vi "test Get and Set RX Start Time.vi"(8 "error in (no error)":errorcluster, 11 "TestCase in":refnum<class "Framework Status Tests.lvclass">) -> (0 "error out":errorcluster, 3 "TestCase out":refnum<class "Framework Status Tests.lvclass">)   [LabVIEW 2017, in "Framework Status Tests.lvclass"]
uses:
  Framework Status Tests.lvclass
  Engine/Classes/Status/Framework Performance.lvclass/Framework Performance.ctl
  <vilib>/addons/_JKI Toolkits/VI Tester/TestCase.llb/TestCase.lvclass
  Engine/Classes/Status/Framework Performance.lvclass
  C:/Program Files (x86)/National Instruments/LabVIEW 2017/vi.lib/addons/_JKI Toolkits/VI Tester/TestCase.llb/TestCase.lvclass
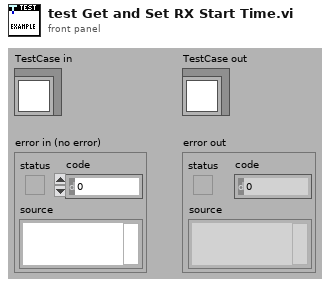
[diagram p1: front panel]
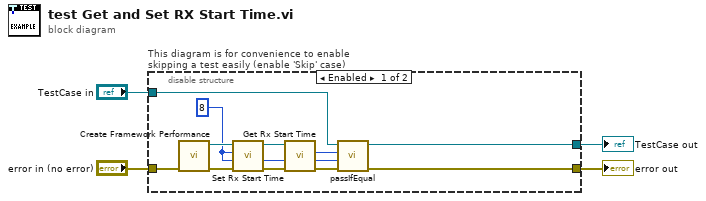
[diagram p0: block diagram]
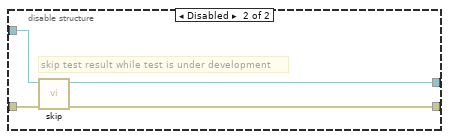
[diagram p2: hidden frame]
diagram:
  n1 = disable-structure "This diagram is for convenience to enable skipping a test easily (enable 'Skip' case)" shown="Enabled" {
    disable-tunnel: "TestCase in" -> [w11 w17]
    disable-tunnel: [w5 w15] -> w1
    disable-tunnel: [w6 w16] -> w3
    disable-tunnel: "error in (no error)" -> [w10 w14]
    frame Enabled {
      w7 = u32 8 ("Rx start time")
      n2 = call "Create Framework Performance.vi"("error in (no error)"=w10) -> ("error out"=w9:errorcluster, "Framework Performance"=w13:refnum<class "Framework Performance.lvclass">)  [unwired: 9 in]
      n3 = call "Set Rx Start Time.vi"("Rx start time"=w7, "Framework Performance in"=w13) -> ("Framework Performance out"=w12:refnum<class "Framework Performance.lvclass">)  [unwired: 9 in]
      n4 = call "Get Rx Start Time.vi"("Framework Performance in"=w12) -> ("Rx start time"=w8:u32)  [unwired: 9 in, 1 out]
      n5 = call-dynamic "passIfEqual.vi"("error in (no error)"=w9, "y"=w7, "x"=w8, "TestCase in"=w11) -> ("error out"=w6:errorcluster, "TestCase out"=w5:refnum<class "Framework Status Tests.lvclass">)  [unwired: 6 in]
    }
    frame Disabled {
      # "skip test result while test is under development"
      n6 = call <vilib>:"skip.vi"("error in (no error)"=w14, "TestCase in"=w17) -> ("error out"=w16:errorcluster, "TestCase out"=w15:refnum<class "Framework Status Tests.lvclass">)  [unwired: 8 in]
    }
  }
  "error out" <- w3
  "TestCase out" <- w1
